vi "Read Field - Variant.vi"(7 "field name":string, 8 "error in (no error)":errorcluster, 9 "type code":T1, 10 "value":variant, 11 "PV Data in":refnum<class "PV Data.lvclass">) -> (0 "error out":errorcluster, 1 "type code out":T1, 2 "value out":variant, 3 "PV Data out":refnum<class "PV Data.lvclass">)   [LabVIEW 2020, in "PV Access.lvlib" / "PV Data.lvlib" / "PV Data.lvclass"]
doc: "Leave <B>field name</B> empty to read the whole data structure."
uses:
  PV Data.lvclass
  <vilib>/ErrorRing/Error Ring.xnode
  3e63842f-1b42-44b7-bfbc-53574ae558bd.vi
  0df52538-0c37-4fc1-a2a6-aa64d23bd73e.vi
  ea7cb730-9445-4e63-a674-7488b051f0a2.vi
  ecc6d044-d1d6-4258-b554-93b542f000c4.vi
  f0dd0353-13dc-4229-be36-72f5216b3ba3.vi
  663b7534-5be4-4c26-8693-775dffd107bf.vi
  6d95b702-a3d4-47fa-b99c-6e9c691d9abd.vi
  334379f0-c2c1-4fd4-b37a-a75153a3c3c1.vi
  22215a59-2fe5-468e-8a76-07a567f1422d.vi
  3b673ad6-c2bb-415d-ac32-dac8d0585a62.vi
  4907590c-51dd-452d-854a-3f23d6337043.vi
  91e94b60-106e-4a8f-bb72-5d9817169e6a.vi
  c7390ac7-e1e0-4f30-b90a-9159575d946d.vi
  aaf6655d-cd8e-45f8-b77e-a22837ed21e0.vi
  830d96f2-0dcb-4e12-99cb-9e6dde05f73e.vi
  77dc8c9c-6059-4e17-8748-14fb7ec0ac2f.vi
  a9875d30-4bd9-4a8c-a52c-f68dec12aa6b.vi
  6dbc08b8-92b8-4054-99f1-d97896c52856.vi
  c55a9e90-05cb-4a8a-8098-6274f5663967.vi
  316c9c8d-b543-4ebf-942d-59175514938d.vi
  229b0493-3b28-4ef3-8240-f1556a969e00.vi
  76e9d66a-8186-463b-a0b5-702645c41f9e.vi
  c324c6c0-264f-44f1-9003-e2f03347ce10.vi
  99229403-bf4d-41b1-8e34-2119cf99b534.vi
  60c7cc55-0a77-42d8-819b-5811e97bdf1a.vi
  <userlib>/_OpenG.lib/lvdata/lvdata.llb/openg_variant.lvlib
  Read Field - Boolean.vi
  Read Field - Boolean Array.vi
  Read Field - I8.vi
  Read Field - I8 Array.vi
  Read Field - I16.vi
  Read Field - I16 Array.vi
  Read Field - I32.vi
  Read Field - I32 Array.vi
  Read Field - I64.vi
  Read Field - I64 Array.vi
  Read Field - U8.vi
  Read Field - U8 Array.vi
  Read Field - U16.vi
  Read Field - U16 Array.vi
  Read Field - U32.vi
  Read Field - U32 Array.vi
  Read Field - U64.vi
  Read Field - U64 Array.vi
  Read Field - SGL.vi
  Read Field - DBL.vi
  Read Field - SGL Array.vi
  Read Field - DBL Array.vi
  Read Field - String.vi
  Read Field - String Array.vi
  <vilib>/Utility/error.llb/Error Cluster From Error Code.vi
  Type Code.ctl
  PV Data.lvlib
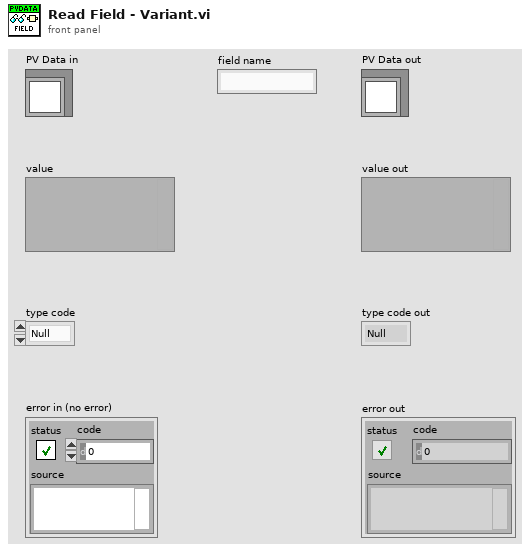
[diagram p1: front panel]
types:
  T1 = typedef "PV Access.lvlib/PV Data.lvlib/Type Code.ctl" = enum8{"Null", "Bool", "BoolA", "Int8", "Int8A", "Int16", "Int16A", "Int32", "Int32A", "Int64", "Int64A", "UInt8", "UInt8A", "UInt16", "UInt16A", "UInt32", "UInt32A", "UInt64", "UInt64A", "Float32", "Float32A", "Float64", "Float64A", "String", "StringA", "Struct", "StructA", "Union", "UnionA", "Any", "AnyA"}
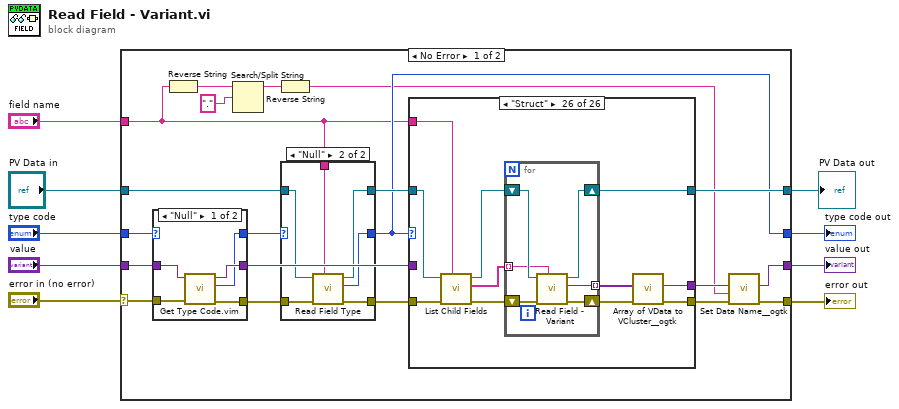
[diagram p0: block diagram]
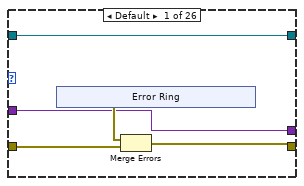
[diagram p4: hidden frame]
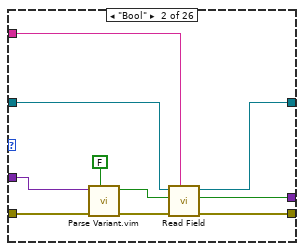
[diagram p5: hidden frame]
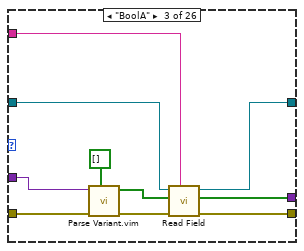
[diagram p6: hidden frame]
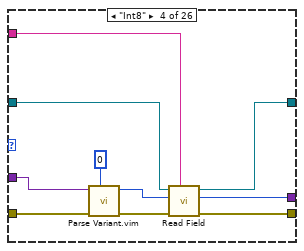
[diagram p7: hidden frame]
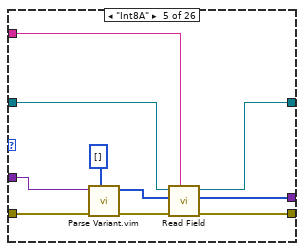
[diagram p8: hidden frame]
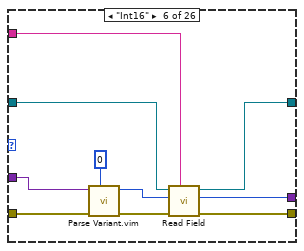
[diagram p9: hidden frame]
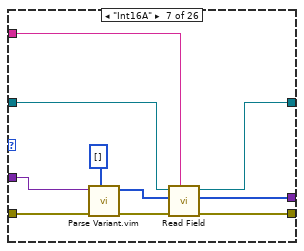
[diagram p10: hidden frame]
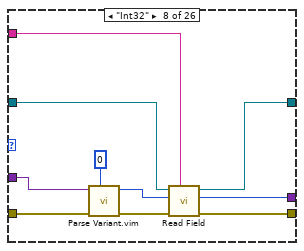
[diagram p11: hidden frame]
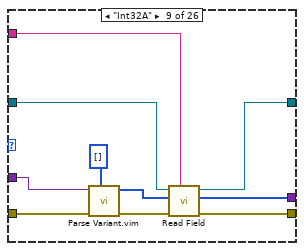
[diagram p12: hidden frame]
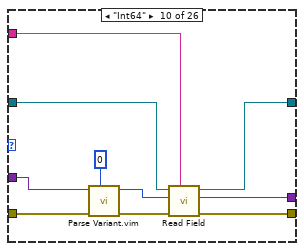
[diagram p13: hidden frame]
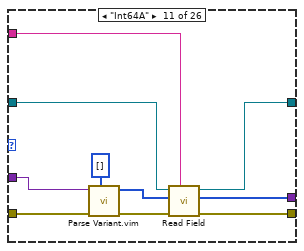
[diagram p14: hidden frame]
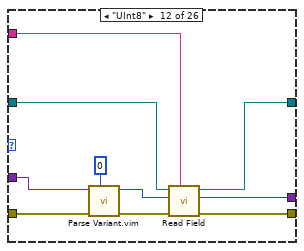
[diagram p15: hidden frame]
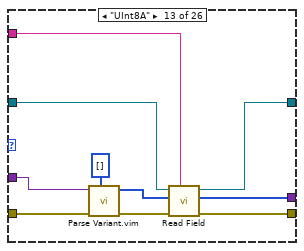
[diagram p16: hidden frame]
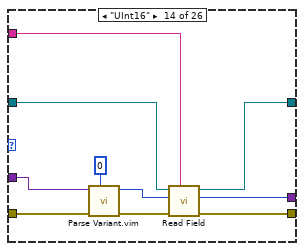
[diagram p17: hidden frame]
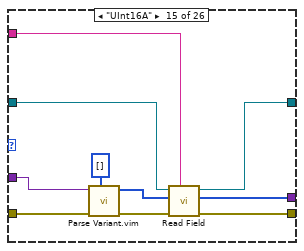
[diagram p18: hidden frame]
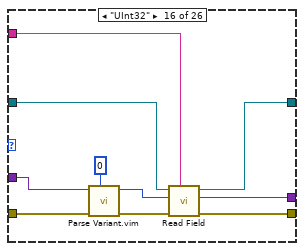
[diagram p19: hidden frame]
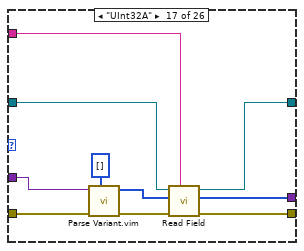
[diagram p20: hidden frame]
diagram:
  n1 = case shown="No Error" "error in (no error)" {
    selector: "error in (no error)" -> [w28 w316]
    tunnel: [w17 w316] -> w8
    tunnel: "PV Data in" -> [w22 w315]
    tunnel: [w29 w315] -> w6
    tunnel: "value" -> [w27 w314]
    tunnel: "type code" -> [w25 w313]
    tunnel: [w15 w314] -> w3
    tunnel: [w19 w313] -> w2
    tunnel: "field name" -> [w11 _]
    frame No Error {
      n2 = case shown="\"Null\"" w25 {
        selector: w25 -> [_ w46]
        tunnel: w28 -> [w43 w45]
        tunnel: [w42 w45] -> w24
        tunnel: w27 -> [w41 w44]
        tunnel: [w40 w44] -> w26
        tunnel: [w39 w46] -> w20
        frame "Null" {
          n3 = call "Get Type Code.vim"("error in"=w43, "value in"=w41) -> ("error out"=w42:errorcluster, "type code"=w39:T1, "value out"=w40:variant)  [unwired: 7 in]
        }
        frame Default {
        }
      }
      n4 = Reverse String(1:w11) -> (0:w13:string)
      n5 = Search/Split String(string=w13, search string/char (-)=".") -> (substring before match=w12:string)  [unwired: 1 in, 2 out]
      n6 = Reverse String(1:w12) -> (0:w10:string)
      n7 = case shown="\"Null\"" w20 {
        selector: w20 -> [w32 _]
        tunnel: w24 -> [w31 w38]
        tunnel: [w31 w37] -> w23
        tunnel: w22 -> [w30 w36]
        tunnel: [w30 w35] -> w21
        tunnel: w11 -> [_ w34]
        tunnel: [w32 w33] -> w19
        frame Default {
        }
        frame "Null" {
          n8 = call "Read Field Type.vi"("field name"=w34, "error in (no error)"=w38, "PV Data in"=w36) -> ("error out"=w37:errorcluster, "type code"=w33:T1, "PV Data out"=w35:refnum<class "PV Data.lvclass">)  [unwired: 6 in]
        }
      }
      n9 = case shown="\"Struct\"" w19 {
        tunnel: [w50 w62 w73 w83 w93 w103 w113 w123 w133 w143 w154 w163 w173 w183 w193 w203 w213 w223 w233 w243 w253 w263 w273 w283 w293 w301] -> w18
        tunnel: w23 -> [w51 w65 w75 w85 w95 w105 w115 w125 w135 w145 w155 w165 w175 w185 w195 w205 w215 w225 w235 w245 w255 w265 w275 w285 w295 w297]
        tunnel: [w48 w60 w71 w82 w91 w101 w111 w121 w131 w141 w152 w161 w171 w182 w191 w201 w212 w221 w231 w241 w251 w261 w271 w281 w291 w303] -> w29
        tunnel: [w47 w59 w69 w80 w89 w99 w109 w119 w129 w139 w150 w159 w169 w180 w189 w199 w210 w219 w229 w239 w249 w259 w269 w279 w289 w299] -> w16
        tunnel: w21 -> [w48 w58 w68 w79 w88 w98 w108 w118 w128 w138 w148 w158 w168 w179 w188 w198 w209 w218 w228 w238 w248 w258 w268 w278 w288 w298]
        tunnel: w26 -> [w47 w57 w66 w76 w86 w96 w106 w116 w126 w136 w146 w156 w166 w176 w186 w196 w206 w216 w226 w236 w246 w256 w266 w276 w286 _]
        tunnel: w11 -> [_ w56 w67 w77 w87 w97 w107 w117 w127 w137 w147 w157 w167 w177 w187 w197 w207 w217 w227 w237 w247 w257 w267 w277 w287 w296]
        frame Default {
          n10 = xnode "Error Ring"() -> ("error out"=w49:errorcluster)
          n11 = Merge Errors(w49, w51) -> (w50:errorcluster)
        }
        frame "Bool" {
          n12 = call "Parse Variant.vim"("default"=FALSE, "error in (no error)"=w65, "value"=w57) -> ("error out"=w63:errorcluster, "value out"=w61:bool)  [unwired: 7 in]
          n13 = call-poly "Read Field.vi"("field name"=w56, "error in (no error)"=w63, "default"=w61, "PV Data in"=w58) -> ("error out"=w62:errorcluster, "value"=w59:bool, "PV Data out"=w60:refnum<class "PV Data.lvclass">)  [unwired: 5 in]
        }
        frame "BoolA" {
          n14 = call "Parse Variant.vim"("default"=bool[] [], "error in (no error)"=w75, "value"=w66) -> ("error out"=w74:errorcluster, "value out"=w72:bool[])  [unwired: 7 in]
          n15 = call-poly "Read Field.vi"("field name"=w67, "error in (no error)"=w74, "default"=w72, "PV Data in"=w68) -> ("error out"=w73:errorcluster, "value"=w69:bool[], "PV Data out"=w71:refnum<class "PV Data.lvclass">)  [unwired: 5 in]
        }
        frame "Int8" {
          n16 = call "Parse Variant.vim"("default"=i8 0, "error in (no error)"=w85, "value"=w76) -> ("error out"=w84:errorcluster, "value out"=w78:i8)  [unwired: 7 in]
          n17 = call-poly "Read Field.vi"("field name"=w77, "error in (no error)"=w84, "default"=w78, "PV Data in"=w79) -> ("error out"=w83:errorcluster, "value"=w80:i8, "PV Data out"=w82:refnum<class "PV Data.lvclass">)  [unwired: 5 in]
        }
        frame "Int8A" {
          n18 = call "Parse Variant.vim"("default"=i8[] [], "error in (no error)"=w95, "value"=w86) -> ("error out"=w94:errorcluster, "value out"=w92:i8[])  [unwired: 7 in]
          n19 = call-poly "Read Field.vi"("field name"=w87, "error in (no error)"=w94, "default"=w92, "PV Data in"=w88) -> ("error out"=w93:errorcluster, "value"=w89:i8[], "PV Data out"=w91:refnum<class "PV Data.lvclass">)  [unwired: 5 in]
        }
        frame "Int16" {
          n20 = call "Parse Variant.vim"("default"=i16 0, "error in (no error)"=w105, "value"=w96) -> ("error out"=w104:errorcluster, "value out"=w102:i16)  [unwired: 7 in]
          n21 = call-poly "Read Field.vi"("field name"=w97, "error in (no error)"=w104, "default"=w102, "PV Data in"=w98) -> ("error out"=w103:errorcluster, "value"=w99:i16, "PV Data out"=w101:refnum<class "PV Data.lvclass">)  [unwired: 5 in]
        }
        frame "Int16A" {
          n22 = call "Parse Variant.vim"("default"=i16[] [], "error in (no error)"=w115, "value"=w106) -> ("error out"=w114:errorcluster, "value out"=w112:i16[])  [unwired: 7 in]
          n23 = call-poly "Read Field.vi"("field name"=w107, "error in (no error)"=w114, "default"=w112, "PV Data in"=w108) -> ("error out"=w113:errorcluster, "value"=w109:i16[], "PV Data out"=w111:refnum<class "PV Data.lvclass">)  [unwired: 5 in]
        }
        frame "Int32" {
          n24 = call "Parse Variant.vim"("default"=0, "error in (no error)"=w125, "value"=w116) -> ("error out"=w124:errorcluster, "value out"=w122:i32)  [unwired: 7 in]
          n25 = call-poly "Read Field.vi"("field name"=w117, "error in (no error)"=w124, "default"=w122, "PV Data in"=w118) -> ("error out"=w123:errorcluster, "value"=w119:i32, "PV Data out"=w121:refnum<class "PV Data.lvclass">)  [unwired: 5 in]
        }
        frame "Int32A" {
          n26 = call "Parse Variant.vim"("default"=i32[] [], "error in (no error)"=w135, "value"=w126) -> ("error out"=w134:errorcluster, "value out"=w132:i32[])  [unwired: 7 in]
          n27 = call-poly "Read Field.vi"("field name"=w127, "error in (no error)"=w134, "default"=w132, "PV Data in"=w128) -> ("error out"=w133:errorcluster, "value"=w129:i32[], "PV Data out"=w131:refnum<class "PV Data.lvclass">)  [unwired: 5 in]
        }
        frame "Int64" {
          n28 = call "Parse Variant.vim"("default"=i64 0, "error in (no error)"=w145, "value"=w136) -> ("error out"=w144:errorcluster, "value out"=w142:i64)  [unwired: 7 in]
          n29 = call-poly "Read Field.vi"("field name"=w137, "error in (no error)"=w144, "default"=w142, "PV Data in"=w138) -> ("error out"=w143:errorcluster, "value"=w139:i64, "PV Data out"=w141:refnum<class "PV Data.lvclass">)  [unwired: 5 in]
        }
        frame "Int64A" {
          n30 = call "Parse Variant.vim"("default"=i64[] [], "error in (no error)"=w155, "value"=w146) -> ("error out"=w149:errorcluster, "value out"=w153:i64[])  [unwired: 7 in]
          n31 = call-poly "Read Field.vi"("field name"=w147, "error in (no error)"=w149, "default"=w153, "PV Data in"=w148) -> ("error out"=w154:errorcluster, "value"=w150:i64[], "PV Data out"=w152:refnum<class "PV Data.lvclass">)  [unwired: 5 in]
        }
        frame "UInt8" {
          n32 = call "Parse Variant.vim"("default"=u8 0, "error in (no error)"=w165, "value"=w156) -> ("error out"=w164:errorcluster, "value out"=w162:u8)  [unwired: 7 in]
          n33 = call-poly "Read Field.vi"("field name"=w157, "error in (no error)"=w164, "default"=w162, "PV Data in"=w158) -> ("error out"=w163:errorcluster, "value"=w159:u8, "PV Data out"=w161:refnum<class "PV Data.lvclass">)  [unwired: 5 in]
        }
        frame "UInt8A" {
          n34 = call "Parse Variant.vim"("default"=u8[] [], "error in (no error)"=w175, "value"=w166) -> ("error out"=w174:errorcluster, "value out"=w172:u8[])  [unwired: 7 in]
          n35 = call-poly "Read Field.vi"("field name"=w167, "error in (no error)"=w174, "default"=w172, "PV Data in"=w168) -> ("error out"=w173:errorcluster, "value"=w169:u8[], "PV Data out"=w171:refnum<class "PV Data.lvclass">)  [unwired: 5 in]
        }
        frame "UInt16" {
          n36 = call "Parse Variant.vim"("default"=u16 0, "error in (no error)"=w185, "value"=w176) -> ("error out"=w184:errorcluster, "value out"=w178:u16)  [unwired: 7 in]
          n37 = call-poly "Read Field.vi"("field name"=w177, "error in (no error)"=w184, "default"=w178, "PV Data in"=w179) -> ("error out"=w183:errorcluster, "value"=w180:u16, "PV Data out"=w182:refnum<class "PV Data.lvclass">)  [unwired: 5 in]
        }
        frame "UInt16A" {
          n38 = call "Parse Variant.vim"("default"=u16[] [], "error in (no error)"=w195, "value"=w186) -> ("error out"=w194:errorcluster, "value out"=w192:u16[])  [unwired: 7 in]
          n39 = call-poly "Read Field.vi"("field name"=w187, "error in (no error)"=w194, "default"=w192, "PV Data in"=w188) -> ("error out"=w193:errorcluster, "value"=w189:u16[], "PV Data out"=w191:refnum<class "PV Data.lvclass">)  [unwired: 5 in]
        }
        frame "UInt32" {
          n40 = call "Parse Variant.vim"("default"=u32 0, "error in (no error)"=w205, "value"=w196) -> ("error out"=w204:errorcluster, "value out"=w202:u32)  [unwired: 7 in]
          n41 = call-poly "Read Field.vi"("field name"=w197, "error in (no error)"=w204, "default"=w202, "PV Data in"=w198) -> ("error out"=w203:errorcluster, "value"=w199:u32, "PV Data out"=w201:refnum<class "PV Data.lvclass">)  [unwired: 5 in]
        }
        frame "UInt32A" {
          n42 = call "Parse Variant.vim"("default"=u32[] [], "error in (no error)"=w215, "value"=w206) -> ("error out"=w214:errorcluster, "value out"=w208:u32[])  [unwired: 7 in]
          n43 = call-poly "Read Field.vi"("field name"=w207, "error in (no error)"=w214, "default"=w208, "PV Data in"=w209) -> ("error out"=w213:errorcluster, "value"=w210:u32[], "PV Data out"=w212:refnum<class "PV Data.lvclass">)  [unwired: 5 in]
        }
        frame "UInt64" {
          n44 = call "Parse Variant.vim"("default"=u64 0, "error in (no error)"=w225, "value"=w216) -> ("error out"=w224:errorcluster, "value out"=w222:u64)  [unwired: 7 in]
          n45 = call-poly "Read Field.vi"("field name"=w217, "error in (no error)"=w224, "default"=w222, "PV Data in"=w218) -> ("error out"=w223:errorcluster, "value"=w219:u64, "PV Data out"=w221:refnum<class "PV Data.lvclass">)  [unwired: 5 in]
        }
        frame "UInt64A" {
          n46 = call "Parse Variant.vim"("default"=u64[] [], "error in (no error)"=w235, "value"=w226) -> ("error out"=w234:errorcluster, "value out"=w232:u64[])  [unwired: 7 in]
          n47 = call-poly "Read Field.vi"("field name"=w227, "error in (no error)"=w234, "default"=w232, "PV Data in"=w228) -> ("error out"=w233:errorcluster, "value"=w229:u64[], "PV Data out"=w231:refnum<class "PV Data.lvclass">)  [unwired: 5 in]
        }
        frame "Float32" {
          n48 = call "Parse Variant.vim"("default"=sgl 0.0, "error in (no error)"=w245, "value"=w236) -> ("error out"=w244:errorcluster, "value out"=w242:sgl)  [unwired: 7 in]
          n49 = call-poly "Read Field.vi"("field name"=w237, "error in (no error)"=w244, "default"=w242, "PV Data in"=w238) -> ("error out"=w243:errorcluster, "value"=w239:sgl, "PV Data out"=w241:refnum<class "PV Data.lvclass">)  [unwired: 5 in]
        }
        frame "Float64" {
          n50 = call "Parse Variant.vim"("default"=0.0, "error in (no error)"=w255, "value"=w246) -> ("error out"=w254:errorcluster, "value out"=w252:dbl)  [unwired: 7 in]
          n51 = call-poly "Read Field.vi"("field name"=w247, "error in (no error)"=w254, "default"=w252, "PV Data in"=w248) -> ("error out"=w253:errorcluster, "value"=w249:dbl, "PV Data out"=w251:refnum<class "PV Data.lvclass">)  [unwired: 5 in]
        }
        frame "Float32A" {
          n52 = call "Parse Variant.vim"("default"=sgl[] [], "error in (no error)"=w265, "value"=w256) -> ("error out"=w264:errorcluster, "value out"=w262:sgl[])  [unwired: 7 in]
          n53 = call-poly "Read Field.vi"("field name"=w257, "error in (no error)"=w264, "default"=w262, "PV Data in"=w258) -> ("error out"=w263:errorcluster, "value"=w259:sgl[], "PV Data out"=w261:refnum<class "PV Data.lvclass">)  [unwired: 5 in]
        }
        frame "Float64A" {
          n54 = call "Parse Variant.vim"("default"=dbl[] [], "error in (no error)"=w275, "value"=w266) -> ("error out"=w274:errorcluster, "value out"=w272:dbl[])  [unwired: 7 in]
          n55 = call-poly "Read Field.vi"("field name"=w267, "error in (no error)"=w274, "default"=w272, "PV Data in"=w268) -> ("error out"=w273:errorcluster, "value"=w269:dbl[], "PV Data out"=w271:refnum<class "PV Data.lvclass">)  [unwired: 5 in]
        }
        frame "String" {
          n56 = call "Parse Variant.vim"("default"="", "error in (no error)"=w285, "value"=w276) -> ("error out"=w284:errorcluster, "value out"=w282:string)  [unwired: 7 in]
          n57 = call-poly "Read Field.vi"("field name"=w277, "error in (no error)"=w284, "default"=w282, "PV Data in"=w278) -> ("error out"=w283:errorcluster, "value"=w279:string, "PV Data out"=w281:refnum<class "PV Data.lvclass">)  [unwired: 5 in]
        }
        frame "StringA" {
          n58 = call "Parse Variant.vim"("default"=string[] [], "error in (no error)"=w295, "value"=w286) -> ("error out"=w294:errorcluster, "value out"=w292:string[])  [unwired: 7 in]
          n59 = call-poly "Read Field.vi"("field name"=w287, "error in (no error)"=w294, "default"=w292, "PV Data in"=w288) -> ("error out"=w293:errorcluster, "value"=w289:string[], "PV Data out"=w291:refnum<class "PV Data.lvclass">)  [unwired: 5 in]
        }
        frame "Struct" {
          n60 = call "List Child Fields.vi"("field name"=w296, "error in (no error)"=w297, "PV Data in"=w298) -> ("error out"=w306:errorcluster, "field names"=w305:string[], "PV Data out"=w304:refnum<class "PV Data.lvclass">)  [unwired: 6 in]
          n61 = for {
            shift-right: [w309] -> w302
            shift-left: w306 -> [w312]
            tunnel: w305 -> [w307] mode=indexing
            shift-right: [w311] -> w303
            shift-left: w304 -> [w310]
            tunnel: [w308] -> w300 mode=indexing
            n62 = call "Read Field - Variant.vi"("field name"=w307, "error in (no error)"=w312, "PV Data in"=w310) -> ("error out"=w309:errorcluster, "value out"=w308:variant, "PV Data out"=w311:refnum<class "PV Data.lvclass">)  [unwired: 5 in, 1 out]
          }
          n63 = call <userlib>:"Array of VData to VCluster__ogtk.vi"("error in (no error)"=w302, "Array"=w300) -> ("error out"=w301:errorcluster, "VCluster"=w299:variant)  [unwired: 8 in]
        }
      }
      n64 = call <userlib>:"Set Data Name__ogtk.vi"("error in (no error)"=w18, "Data Name"=w10, "Data"=w16) -> ("error out"=w17:errorcluster, "Renamed Data"=w15:variant)  [unwired: 7 in]
    }
    frame Error {
    }
  }
  "value out" <- w3
  "error out" <- w8
  "PV Data out" <- w6
  "type code out" <- w2
